vi "HMS_Firmware_Manager_II_Scan.vi"(11 "error in (no error)":errorcluster) -> (4 "standard error":string="\r\n", 6 "standard output":string, 8 "PASS?":bool, 10 "Module Detected":bool, 15 "error out":errorcluster)   [LabVIEW 2025]
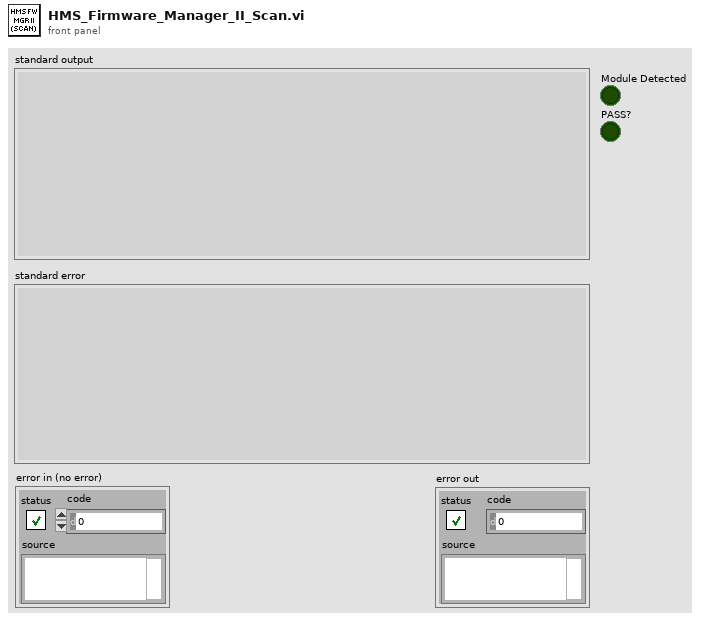
[diagram p1: front panel]
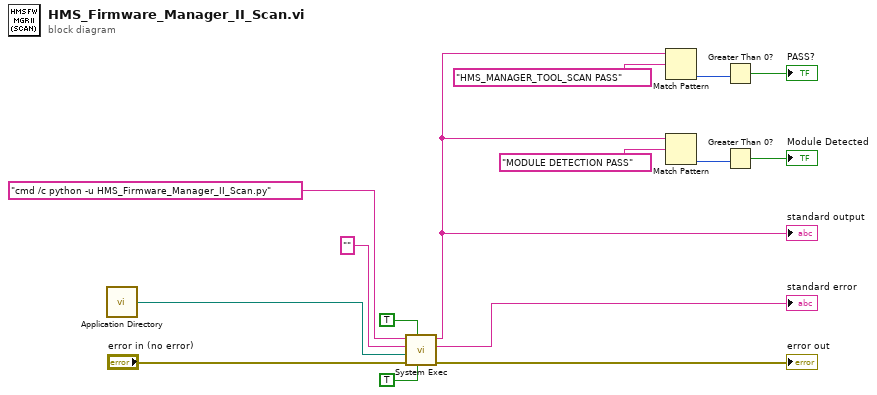
[diagram p0: block diagram]
diagram:
  n1 = call <vilib>:"Application Directory.vi"() -> ("Application Directory"=w1:path)
  n2 = call <vilib>:"System Exec.vi"("run minimized? (F)"=TRUE, "wait until completion? (T)"=TRUE ("run minimized? (F)"), "error in (no error)"="error in (no error)", "working directory"=w1, "standard input"="", "command line"="cmd /c python -u HMS_Firmware_Manager_II_Scan.py" ("name or relative path")) -> ("error out"=→"error out":errorcluster, "standard error"=→"standard error":string, "standard output"=w2:string)  [unwired: 2 in, 1 out]
  "standard output" <- w2
  n3 = Match Pattern(string=w2, regular expression="HMS_MANAGER_TOOL_SCAN PASS") -> (offset past match=w5:i32)  [unwired: 1 in, 3 out]
  n4 = Match Pattern(string=w2, regular expression="MODULE DETECTION PASS") -> (offset past match=w8:i32)  [unwired: 1 in, 3 out]
  n5 = Greater Than 0?(x=w5) -> (x > 0?=→"PASS?":bool)
  n6 = Greater Than 0?(x=w8) -> (x > 0?=→"Module Detected":bool)
